vi "make_probe_point_headers.vi"() -> ()   [LabVIEW 2012]
uses:
  probe_point.ctl
  initialization/micron_globals.vi
panel:
  out "probe_points.h":path
  out "probe_points.m":path
  # "This VI is used to generate the probe_points.m and probe_points.h files when the trace data format changes (defined by probe_points.ctl, status_flag.ctl, \"Trace data version\". )  These files are written into the labview source tree (where this VI is located.)   All you have to do is run this VI on the windows host."
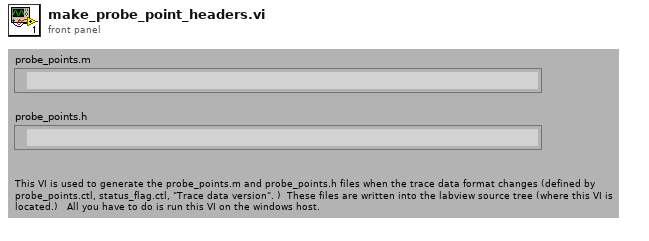
[diagram p1: front panel]
types:
  T1 = typedef "probe_point.ctl" = enum16{"Position (tip)", "Position (RCM)", "Null pos (tip)", "Null pos (RCM)", "V limiter (tip)", "V Limiter (RCM)", "Goal (tip)", "Goal (RCM)", "Link pos 0", "Link pos 1", "KF link pos 0", "KF link pos 1", "Link rate 0", "Link rate 1", "Link residue 0", "Link residue 1", "Link goal 0", "Link goal 1", "Rate limit 0", "Rate limit 1", "Link error 0", "Link error 1", "Controller 0", "Controller 1", "Output 0", "Output 1", "Drive 0", "Drive 1", "Stimulus 0", "Stimulus 1", "Trace data 0", "Trace data 1", "Analog data 0", "Analog data 1", "Status flags", "Light 0", "Light 1", "Light 2", "Light 3", "Light 4", "Light 5", "Goal origin", "Goal rotation 0", "Goal rotation 1", "Goal rotation 2", "Output origin", "Output rotation 0", "Output rotation 1", "Output rotation 2", "Handle origin", "Handle rotation 0", "Handle rotation 1", "Handle rotation 2", "Handle position", "Handle velocity", "Handle acceleration", "Handle angles", "Handle angle rates", "Handle pos residue", "Handle angle residue", "Trace length"}
  T2 = enum16{"open", "replace", "create", "open or create", "replace or create", "replace or create with confirmation"}
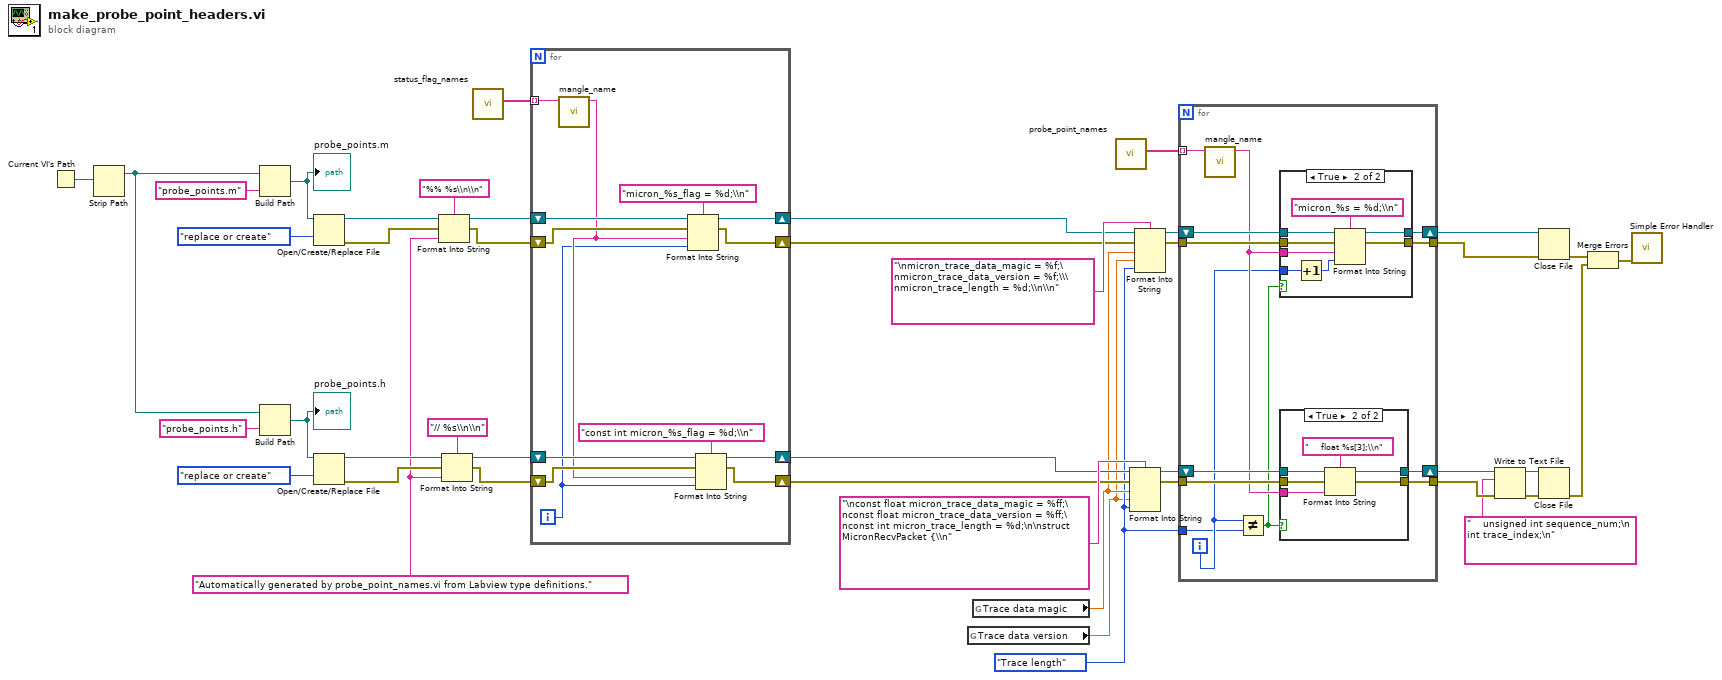
[diagram p0: block diagram]
diagram:
  w7 = "Automatically generated by probe_point_names.vi from Labview type definitions." ("text")
  w2 = probe_point."Trace length" ("Probe point")
  n1 = Current VI's Path() -> (path=w41:path)
  n2 = Strip Path(path=w41) -> (stripped path=w26:path)  [unwired: 1 out]
  n3 = Build Path(base path=w26, name or relative path="probe_points.m" ("replace string (\"\")")) -> (appended path=w43:path)
  "probe_points.m" <- w43
  n4 = Build Path(base path=w26, name or relative path="probe_points.h" ("replace string (\"\")")) -> (appended path=w34:path)
  "probe_points.h" <- w34
  n5 = Open/Create/Replace File(file path (use dialog)=w43, operation (0:open)=T2."replace or create") -> (refnum out=w14:refnum<file>, error out=w13:errorcluster)  [unwired: 4 in, 1 out]
  n6 = Open/Create/Replace File(file path (use dialog)=w34, operation (0:open)=T2."replace or create") -> (refnum out=w9:refnum<file>, error out=w8:errorcluster)  [unwired: 4 in, 1 out]
  n7 = Format Into String(format string="%% %s\\n\\n", initial string=w14, error in=w13, w7) -> (resulting string=w12:refnum<file>, error out=w11:errorcluster)
  n8 = Format Into String(format string="// %s\\n\\n", initial string=w9, error in=w8, w7) -> (resulting string=w6:refnum<file>, error out=w4:errorcluster)
  n9 = call "status_flag_names.vi"() -> ("Names"=w15:string[])  [unwired: 11 in]
  n10 = for {
    shift-right: [w53] -> w19
    shift-left: w12 -> [w55]
    shift-right: [w52] -> w18
    shift-left: w11 -> [w54]
    shift-right: [w48] -> w16
    shift-left: w6 -> [w50]
    shift-right: [w47] -> w17
    shift-left: w4 -> [w49]
    tunnel: w15 -> [w57] mode=indexing
    i -> [w45]
    n11 = call "mangle_name.vi"("String in"=w57) -> ("String out"=w46:string)  [unwired: 10 in]
    n12 = Format Into String(format string="micron_%s_flag = %d;\\n", initial string=w55, error in=w54, w46, w45) -> (resulting string=w53:refnum<file>, error out=w52:errorcluster)
    n13 = Format Into String(format string="const int micron_%s_flag = %d;\\n", initial string=w50, error in=w49, w46, w45) -> (resulting string=w48:refnum<file>, error out=w47:errorcluster)
  }
  n14 = global read "micron_globals.vi" "Trace data version"() -> (w1:sgl)
  n15 = global read "micron_globals.vi" "Trace data magic"() -> (w3:sgl)
  n16 = call "probe_point_names.vi"() -> ("Names"=w20:string[])  [unwired: 11 in]
  n17 = Format Into String(format string="\nconst float micron_trace_data_magic = %ff;\nconst float micron_trace_data_version = %ff;\nconst int micron_trace_length = %d;\n\nstruct MicronRecvPacket {\\n", initial string=w16, error in=w17, w3, w1, w2) -> (resulting string=w38:refnum<file>, error out=w37:errorcluster)
  n18 = Format Into String(format string="\nmicron_trace_data_magic = %f;\nmicron_trace_data_version = %f;\\\nmicron_trace_length = %d;\\n\\n", initial string=w19, error in=w18, w3, w1, w2) -> (resulting string=w32:refnum<file>, error out=w31:errorcluster)
  n19 = for {
    tunnel: w20 -> [w69] mode=indexing
    tunnel: w31 -> [w67]
    tunnel: [w66] -> w39
    shift-right: [w68] -> w40
    shift-left: w32 -> [w70]
    tunnel: w37 -> [w64]
    tunnel: [w65] -> w24
    shift-right: [w63] -> w25
    shift-left: w38 -> [w62]
    tunnel: w2 -> [w59]
    i -> [w60]
    n20 = call "mangle_name.vi"("String in"=w69) -> ("String out"=w61:string)  [unwired: 10 in]
    n21 = Not Equal?(x=w60, y=w59) -> (x != y?=w58:bool)
    n22 = case shown="True" w58 {
      tunnel: w70 -> [w72 w80]
      tunnel: [w72 w77] -> w68
      tunnel: w67 -> [w71 w76]
      tunnel: [w71 w75] -> w66
      tunnel: w61 -> [_ w74]
      tunnel: w60 -> [_ w73]
      frame False {
      }
      frame True {
        n23 = Increment(x=w73) -> (x+1=w78:i32)
        n24 = Format Into String(format string="micron_%s = %d;\\n", initial string=w80, error in=w76, w74, w78) -> (resulting string=w77:refnum<file>, error out=w75:errorcluster)
      }
    }
    n25 = case shown="True" w58 {
      tunnel: [w81 w88] -> w65
      tunnel: w64 -> [w81 w87]
      tunnel: [w82 w86] -> w63
      tunnel: w62 -> [w82 w84]
      tunnel: w61 -> [_ w83]
      frame False {
      }
      frame True {
        n26 = Format Into String(format string="    float %s[3];\\n", initial string=w84, error in=w87, w83) -> (resulting string=w86:refnum<file>, error out=w88:errorcluster)
      }
    }
  }
  n27 = Write to Text File(file (use dialog)=w25, text="    unsigned int sequence_num;\n    int trace_index;\n", error in=w24) -> (refnum out=w22:refnum<file>, error out=w21:errorcluster)  [unwired: 1 in, 1 out]
  n28 = Close File(refnum=w40, error in=w39) -> (error out=w29:errorcluster)  [unwired: 1 out]
  n29 = Close File(refnum=w22, error in=w21) -> (error out=w28:errorcluster)  [unwired: 1 out]
  n30 = Merge Errors(w29, w28) -> (w27:errorcluster)
  n31 = call <vilib>:"Simple Error Handler.vi"("error in (no error)"=w27) -> ()  [unwired: 4 in, 5 out]
